vi "configure runtime data.vi"(4 "output dictionary":refnum<class "data dictionary.lvclass">, 6 "input dictionary":refnum<class "data dictionary.lvclass">, 8 "error in":errorcluster, 10 "Slave Info List":T6(array[cluster]), 11 "Profibus Module configuration in":refnum<class "Profibus Module configuration.lvclass">) -> (0 "error out":errorcluster, 1 "diagnostics":T1[](array[typedef]), 2 "inputs":T3[](array[typedef]), 3 "outputs":T3[](array[typedef]))   [LabVIEW 2013, in "Profibus Module runtime.lvclass"]
uses:
  Profibus Module runtime.lvclass
  configuration/Profibus Module configuration.lvclass
  profibus slave configuration.ctl
  profibus mapping configuration.ctl
  <vilib>/NI/Tag Bus/tag/Data Type.ctl
  <vilib>/NI/Tag Bus/dictionary/data dictionary.lvclass
  profibus diagnostics reporting.ctl
  configuration/error throw specification.ctl
  configuration/Profibus Module configuration.lvclass/Profibus Module configuration.ctl
  channel/Profibus channel.lvclass/Profibus channel.ctl
  <vilib>/NI/Tag Bus Module Framework/channel/TBM channel.lvclass/TBM channel.ctl
  <vilib>/NI/Tag Bus/tag/tag descriptor.lvclass/tag descriptor.ctl
  <vilib>/NI/Tag Bus/dictionary/data dictionary.lvclass/data dictionary.ctl
  configuration/Read slave diagnostics.vi
  <vilib>/NI/Tag Bus/dictionary/look up tag by type.vi
  <vilib>/NI/Tag Bus/dictionary/lookup polymorphs/locate Array of U8.vi
  <vilib>/NI/Tag Bus/dictionary/search/find data index.vi
  <vilib>/NI/Tag Bus/dictionary/search/search string list.vi
  <vilib>/NI/Tag Bus/dictionary/tag not found.vi
  <vilib>/NI/Tag Bus/tag/tag descriptor.lvclass
  <vilib>/NI/Tag Bus Module Framework/channel/TBM channel.lvclass
  channel/Profibus channel.lvclass
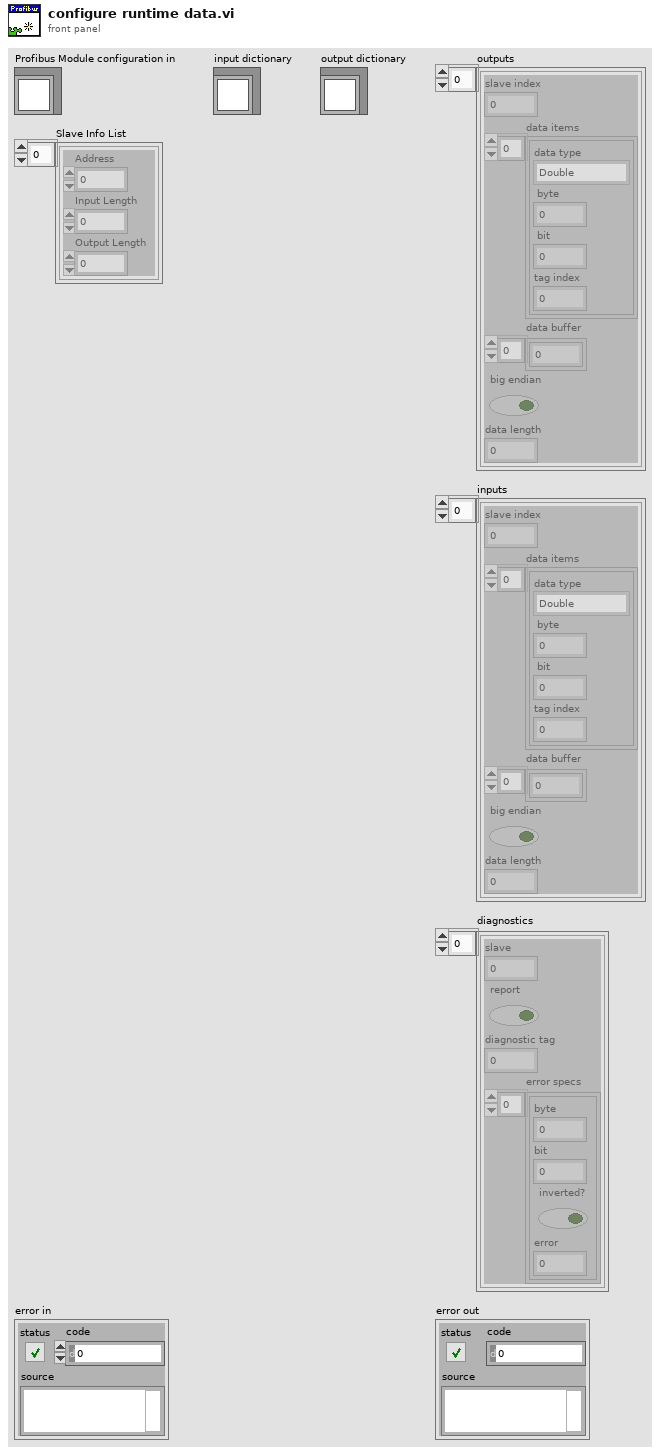
[diagram p1: front panel]
types:
  T1 = typedef "Profibus Module runtime.lvclass/profibus diagnostics reporting.ctl" = cluster{"slave":i8, "report":bool, "diagnostic tag":i32, "error specs":T2[]}
  T2 = typedef "Profibus Module configuration.lvclass/error throw specification.ctl" = cluster{"byte":i32, "bit":i32, "inverted?":bool, "error":i32}
  T3 = typedef "Profibus Module runtime.lvclass/profibus slave configuration.ctl" = cluster{"slave index":i8, "data items":T4[], "data buffer":u8[], "big endian":bool, "data length":i32}
  T4 = typedef "Profibus Module runtime.lvclass/profibus mapping configuration.ctl" = cluster{"data type":T5, " byte":i32, " bit":i32, "tag index":i32}
  T5 = typedef "tag bus.lvlib/tag descriptor.lvclass/Data Type.ctl" = enum16{"Double", "Single", "I64", "I32", "I16", "I8", "U64", "U32", "U16", "U8", "Boolean", "String", "Array of Double", "Array of Single", "Array of I64", "Array of I32", "Array of I16", "Array of I8", "Array of U64", "Array of U32", "Array of U16", "Array of U8", "Array of Boolean", "Array of String"}
  T6 = cluster{"Address":i8, "Input Length":u8, "Output Length":u8}[]
  T7 = typedef "Profibus Module configuration.lvclass/endianness setting.ctl" = cluster{"slave":i8, "big endian":bool}
  T8 = typedef "TBM channel.lvclass/channel classification.ctl" = enum16{"input data", "output data", "processing parameter", "processing result"}
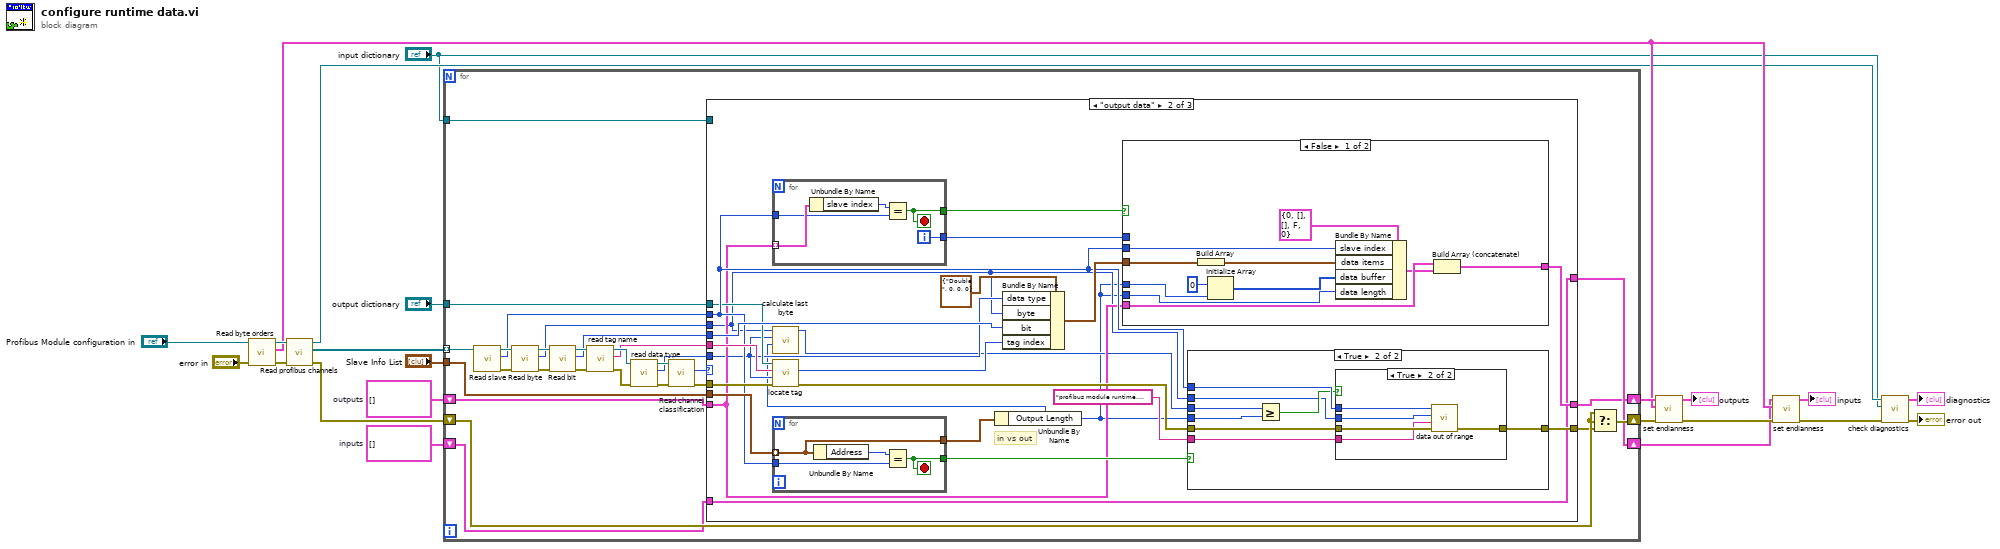
[diagram p0: block diagram]
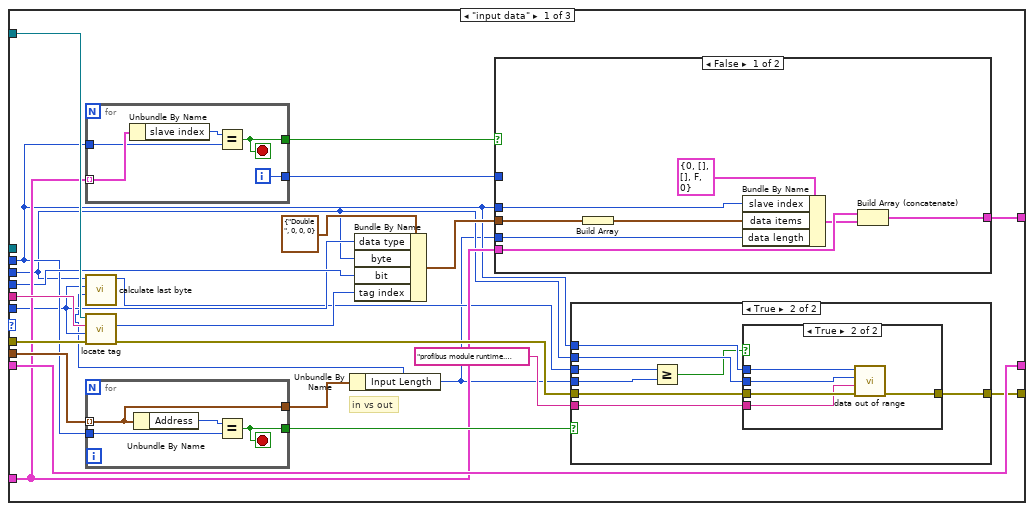
[diagram p2: hidden frame]
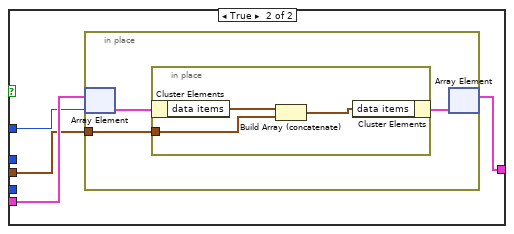
[diagram p3: hidden frame]
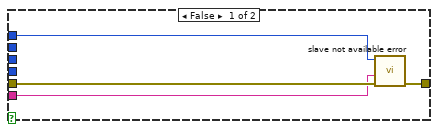
[diagram p4: hidden frame]
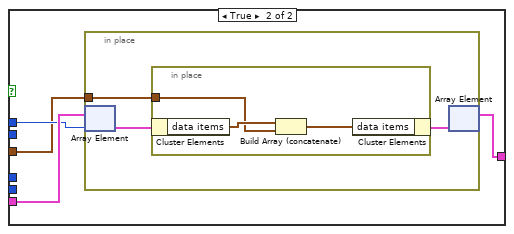
[diagram p6: hidden frame]
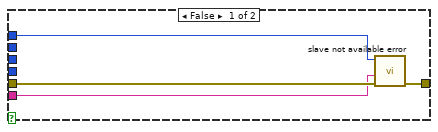
[diagram p7: hidden frame]
diagram:
  w19 = T3[] []  # outputs
  w20 = T3[] []  # inputs
  n1 = call "Read byte orders.vi"("error in"="error in", "Profibus Module configuration in"="Profibus Module configuration in") -> ("error out"=w14:errorcluster, "byte orders"=w8:T7[], "Profibus Module configuration out"=w15:refnum<class "Profibus Module configuration.lvclass">)  [unwired: 7 in]
  n2 = call "Read profibus channels.vi"("error in"=w14, "Profibus Module configuration in"=w15) -> ("error out"=w22:errorcluster, "channels"=w21:refnum<class "Profibus channel.lvclass">[], "Profibus Module configuration out"=w2:refnum<class "Profibus Module configuration.lvclass">)  [unwired: 7 in]
  n3 = for {
    shift-right: [w49] -> w11
    shift-left: w22 -> [w50]
    tunnel: w21 -> [w32] mode=indexing
    shift-right: [w45] -> w7
    shift-left: w20 -> [w44]
    shift-right: [w43] -> w12
    shift-left: w19 -> [w42]
    tunnel: "Slave Info List" -> [w46]
    tunnel: "input dictionary" -> [w48]
    tunnel: "output dictionary" -> [w47]
    n4 = call "Read slave.vi"("Profibus channel in"=w32) -> ("error out"=w29:errorcluster, "slave"=w25:i8, "Profibus channel out"=w30:refnum<class "Profibus channel.lvclass">)  [unwired: 8 in]
    n5 = call "Read byte.vi"("error in"=w29, "Profibus channel in"=w30) -> ("error out"=w28:errorcluster, "byte"=w24:i32, "Profibus channel out"=w31:refnum<class "Profibus channel.lvclass">)  [unwired: 7 in]
    n6 = call "Read bit.vi"("error in"=w28, "Profibus channel in"=w31) -> ("error out"=w27:errorcluster, "bit"=w23:i32, "Profibus channel out"=w26:refnum<class "Profibus channel.lvclass">)  [unwired: 7 in]
    n7 = call <vilib>:"read tag name.vi"("error in"=w27, "system tag in"=w26) -> ("error out"=w37:errorcluster, "name"=w38:string, "system tag out"=w40:refnum<class "Profibus channel.lvclass">)  [unwired: 7 in]
    n8 = call <vilib>:"read data type.vi"("error in"=w37, "system tag in"=w40) -> ("error out"=w35:errorcluster, "data type"=w36:T5, "system tag out"=w39:refnum<class "Profibus channel.lvclass">)  [unwired: 7 in]
    n9 = call <vilib>:"Read channel classification.vi"("error in"=w35, "channel in"=w39) -> ("error out"=w34:errorcluster, "channel classification"=w33:T8)  [unwired: 7 in, 1 out]
    n10 = case shown="\"output data\"" w33 {
      tunnel: w34 -> [w72 w141 w190]
      tunnel: w36 -> [w54 w122 _]
      tunnel: w48 -> [w70 _ _]
      tunnel: w47 -> [_ w126 _]
      tunnel: w46 -> [w69 w139 _]
      tunnel: [w60 w123 w192] -> w45
      tunnel: w44 -> [w61 w123 w192]
      tunnel: [w73 w124 w191] -> w43
      tunnel: w42 -> [w73 w125 w191]
      tunnel: [w67 w137 w190] -> w41
      tunnel: w25 -> [w55 w127 _]
      tunnel: w24 -> [w53 w121 _]
      tunnel: w23 -> [w57 w129 _]
      tunnel: w38 -> [w71 w140 _]
      frame "input data" {
        # "in vs out"
        n11 = for {
          tunnel: w61 -> [w118] mode=indexing
          tunnel: w55 -> [w116]
          tunnel: [w115] -> w63
          tunnel: [w114] -> w62
          i -> [w114]
          stop <- w115 stop-if-true
          n12 = Unbundle By Name(w118) -> ("slave index"=w117:i8)
          n13 = Equal?(x=w117, y=w116) -> (x = y?=w115:bool)
        }
        n14 = call <vilib>:"locate tag.vi"("error in"=w72, "data type"=w54, "name"=w71, "data dictionary in"=w70) -> ("error out"=w68:errorcluster, "index"=w56:i32)  [unwired: 5 in, 1 out]
        n15 = for {
          tunnel: w69 -> [w110] mode=indexing
          tunnel: w55 -> [w112]
          tunnel: [w111] -> w66
          tunnel: [w110] -> w65
          stop <- w111 stop-if-true
          n16 = Unbundle By Name(w110) -> ("Address"=w113:i8)
          n17 = Equal?(x=w113, y=w112) -> (x = y?=w111:bool)
        }
        n18 = Unbundle By Name(w65) -> ("Input Length"=w51:u8)
        n19 = call "calculate last byte.vi"("Input Length"=w51, "type"=w54, "byte in"=w53) -> ("last byte"=w52:i32)  [unwired: 8 in]
        n20 = Bundle By Name(cluster=T4 {"data type"=enum."Double", " byte"=0, " bit"=0, "tag index"=0} ("data items"), "data type"=w54, "byte"=w53, "bit"=w57, "tag index"=w56) -> (w58:T4)
        n21 = case shown="False" w63 {
          tunnel: w62 -> [_ w84]
          tunnel: w61 -> [w81 w85]
          tunnel: [w80 w83] -> w60
          tunnel: w58 -> [w77 w82]
          tunnel: w55 -> [w75 _]
          tunnel: w51 -> [w74 _]
          frame False {
            n22 = Build Array(w77) -> (w76:T4[])
            n23 = Bundle By Name(cluster=T3 {"slave index"=0, "data items"=[], "data buffer"=[], "big endian"=FALSE, "data length"=0} ("slave configuration"), "slave index"=w75, "data items"=w76, "data length"=w74) -> (w78:T3)
            n24 = Build Array (concatenate)(w81, w78) -> (w80:T3[])
          }
          frame True {
            n25 = in-place {
              in-place-border: w82 -> [w86]
              n26 = in-place-array #1(w85, w84) -> (w88:T3)
              n27 = in-place {
                in-place-border: w86 -> [w89]
                n28 = in-place-cluster #2(w88) -> ("data items"=w91:T4[])
                n29 = Build Array (concatenate)(w91, w89) -> (w90:T4[])
                n30 = in-place-cluster #2("data items"=w90) -> (w87:T3)
              }
              n31 = in-place-array #1(w87) -> (w83:T3[])  [unwired: 1 out]
            }
          }
        }
        n32 = case shown="True" w66 {
          tunnel: w68 -> [w95 w102]
          tunnel: [w94 w103] -> w67
          tunnel: w55 -> [w93 w99]
          tunnel: w51 -> [_ w100]
          tunnel: w53 -> [_ w98]
          tunnel: "profibus module runtime.lvclass>>init.vi>>configure runtime data.vi" ("source") -> [w92 w101]
          tunnel: w52 -> [_ w96]
          frame False {
            n33 = call "slave not available error.vi"("error in"=w95, "source"=w92, "slave"=w93) -> ("error out"=w94:errorcluster)  [unwired: 8 in]
          }
          frame True {
            n34 = Greater Or Equal?(x=w96, y=w100) -> (x >= y?=w97:bool)
            n35 = case shown="True" w97 {
              tunnel: [w104 w109] -> w103
              tunnel: w102 -> [w104 w108]
              tunnel: w101 -> [_ w107]
              tunnel: w99 -> [_ w106]
              tunnel: w98 -> [_ w105]
              frame False {
              }
              frame True {
                n36 = call "data out of range.vi"("error in"=w108, "source"=w107, "byte"=w105, "slave"=w106) -> ("error out"=w109:errorcluster)  [unwired: 7 in]
              }
            }
          }
        }
      }
      frame "output data" {
        # "in vs out"
        n37 = for {
          tunnel: w125 -> [w189] mode=indexing
          tunnel: w127 -> [w187]
          tunnel: [w186] -> w133
          tunnel: [w185] -> w132
          i -> [w185]
          stop <- w186 stop-if-true
          n38 = Unbundle By Name(w189) -> ("slave index"=w188:i8)
          n39 = Equal?(x=w188, y=w187) -> (x = y?=w186:bool)
        }
        n40 = call <vilib>:"locate tag.vi"("error in"=w141, "data type"=w122, "name"=w140, "data dictionary in"=w126) -> ("error out"=w138:errorcluster, "index"=w128:i32)  [unwired: 5 in, 1 out]
        n41 = for {
          tunnel: w139 -> [w181] mode=indexing
          tunnel: w127 -> [w183]
          tunnel: [w182] -> w136
          tunnel: [w181] -> w135
          stop <- w182 stop-if-true
          n42 = Unbundle By Name(w181) -> ("Address"=w184:i8)
          n43 = Equal?(x=w184, y=w183) -> (x = y?=w182:bool)
        }
        n44 = Unbundle By Name(w135) -> ("Output Length"=w119:u8)
        n45 = call "calculate last byte.vi"("Input Length"=w119, "type"=w122, "byte in"=w121) -> ("last byte"=w120:i32)  [unwired: 8 in]
        n46 = Bundle By Name(cluster=T4 {"data type"=enum."Double", " byte"=0, " bit"=0, "tag index"=0} ("data items"), "data type"=w122, "byte"=w121, "bit"=w129, "tag index"=w128) -> (w130:T4)
        n47 = case shown="False" w133 {
          tunnel: w132 -> [_ w155]
          tunnel: w125 -> [w152 w156]
          tunnel: [w151 w154] -> w124
          tunnel: w130 -> [w148 w153]
          tunnel: w127 -> [w146 _]
          tunnel: w119 -> [w144 _]
          tunnel: w119 -> [w142 _]
          frame False {
            n48 = Build Array(w148) -> (w147:T4[])
            n49 = Initialize Array(u8 0 ("Numeric"), w144) -> (w143:u8[])
            n50 = Bundle By Name(cluster=T3 {"slave index"=0, "data items"=[], "data buffer"=[], "big endian"=FALSE, "data length"=0} ("slave configuration"), "slave index"=w146, "data items"=w147, "data buffer"=w143, "data length"=w142) -> (w149:T3)
            n51 = Build Array (concatenate)(w152, w149) -> (w151:T3[])
          }
          frame True {
            n52 = in-place {
              in-place-border: w153 -> [w157]
              n53 = in-place-array #3(w156, w155) -> (w159:T3)
              n54 = in-place {
                in-place-border: w157 -> [w160]
                n55 = in-place-cluster #4(w159) -> ("data items"=w162:T4[])
                n56 = Build Array (concatenate)(w162, w160) -> (w161:T4[])
                n57 = in-place-cluster #4("data items"=w161) -> (w158:T3)
              }
              n58 = in-place-array #3(w158) -> (w154:T3[])  [unwired: 1 out]
            }
          }
        }
        n59 = case shown="True" w136 {
          tunnel: w138 -> [w166 w173]
          tunnel: [w165 w174] -> w137
          tunnel: w127 -> [w164 w170]
          tunnel: w119 -> [_ w171]
          tunnel: w121 -> [_ w168]
          tunnel: "profibus module runtime.lvclass>>init.vi>>configure runtime data.vi" ("source") -> [w163 w172]
          tunnel: w120 -> [_ w167]
          frame False {
            n60 = call "slave not available error.vi"("error in"=w166, "source"=w163, "slave"=w164) -> ("error out"=w165:errorcluster)  [unwired: 8 in]
          }
          frame True {
            n61 = Greater Or Equal?(x=w167, y=w171) -> (x >= y?=w169:bool)
            n62 = case shown="True" w169 {
              tunnel: [w175 w180] -> w174
              tunnel: w173 -> [w175 w179]
              tunnel: w172 -> [_ w178]
              tunnel: w170 -> [_ w177]
              tunnel: w168 -> [_ w176]
              frame False {
              }
              frame True {
                n63 = call "data out of range.vi"("error in"=w179, "source"=w178, "byte"=w176, "slave"=w177) -> ("error out"=w180:errorcluster)  [unwired: 7 in]
              }
            }
          }
        }
      }
      frame Default {
      }
    }
    n64 = Select(t=w50, s=w50, f=w41) -> (s? t:f=w49:errorcluster)
  }
  n65 = call "set endianness.vi"("error in"=w11, "byte orders"=w8, "config in"=w12) -> ("error out"=w9:errorcluster, "config out"=→"outputs":T3[])  [unwired: 7 in]
  n66 = call "set endianness.vi"("error in"=w9, "byte orders"=w8, "config in"=w7) -> ("error out"=w4:errorcluster, "config out"=→"inputs":T3[])  [unwired: 7 in]
  n67 = call "check diagnostics.vi"("error in"=w4, "data dictionary in"="input dictionary", "Profibus Module configuration in"=w2) -> ("error out"=→"error out":errorcluster, "diagnostics"=→"diagnostics":T1[])  [unwired: 7 in]
